vi "TCP Wait on Ready.vi"(7 "error in":errorcluster) -> (0 "error out":errorcluster)   [LabVIEW 2013]
panel:
  out "data out":string
  out "Busy?":bool
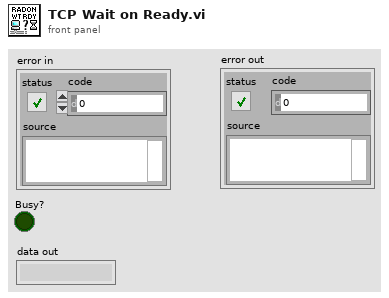
[diagram p1: front panel]
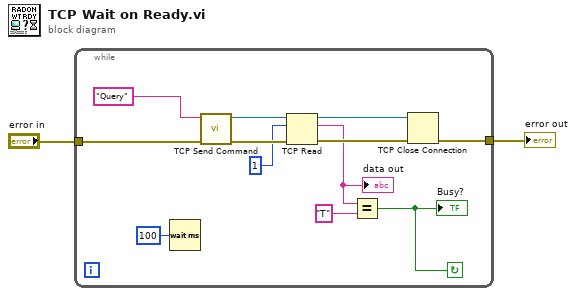
[diagram p0: block diagram]
diagram:
  n1 = while {
    tunnel: "error in" -> [w14]
    tunnel: [w7] -> w1
    stop <- w4 continue-if-true
    n2 = Wait (ms)(milliseconds to wait=u32 100) -> ()  [unwired: 1 out]
    n3 = call "TCP Send Command.vi"("error in"=w14, "Command"="Query") -> ("error out"=w12:errorcluster, "connection ID out"=w11:refnum<k5>)  [unwired: 8 in]
    n4 = TCP Read(connection ID=w11, bytes to read=1, error in (no error)=w12) -> (connection ID out=w8:refnum<k5>, data out=w6:string, error out=w9:errorcluster)  [unwired: 2 in]
    "data out" <- w6
    n5 = Equal?(x=w6, y="T") -> (x = y?=w4:bool)
    "Busy?" <- w4
    n6 = TCP Close Connection(connection ID=w8, error in (no error)=w9) -> (error out=w7:errorcluster)  [unwired: 1 in, 1 out]
  }
  "error out" <- w1
